vi "Front Panel Main Pange Horizontal Scroll Bar.vi"(8 "error in":errorcluster, 9 "Scrollbar Visibility":T1(ring)=enum."Off While Running", 11 "VI Ref In":refnum<vi>) -> (0 "error out":errorcluster, 3 "VI Ref Out":refnum<vi>)   [LabVIEW 2024]
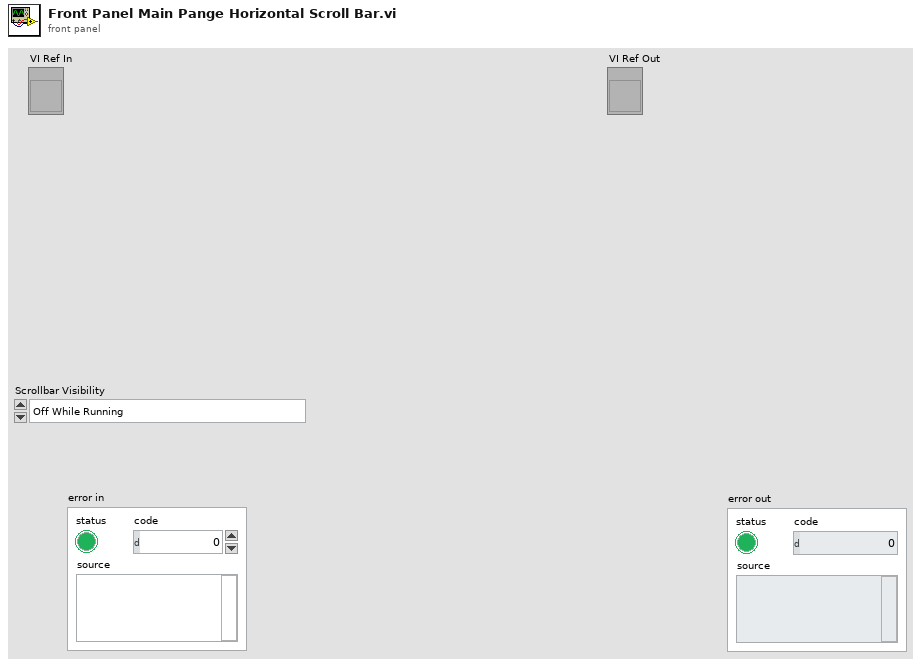
[diagram p1: front panel]
types:
  T1 = enum16{"Always On", "Always Off", "Off While Running"}
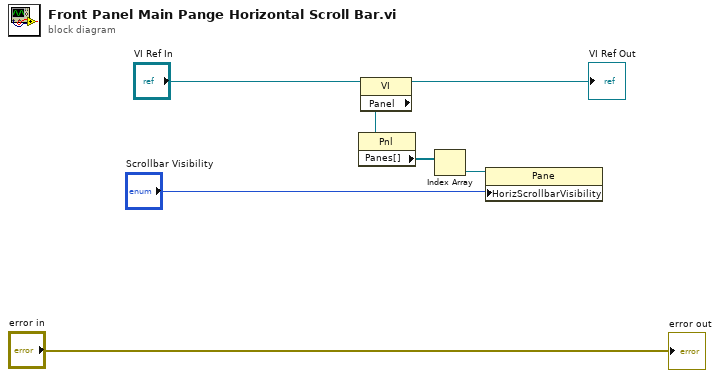
[diagram p0: block diagram]
diagram:
  n1 = property class="VI"(reference="VI Ref In") -> (reference out=→"VI Ref Out":refnum<vi>, "Panel"=w7:refnum<vi>)  [unwired: 1 in, 1 out]
  n2 = property class="Pnl"(reference=w7) -> ("Panes[]"=w6:refnum<vi>[])  [unwired: 1 in, 2 out]
  n3 = Index Array(array=w6) -> (element=w5:refnum<vi>)  [unwired: 1 in]
  n4 = property class="Pane"(reference=w5, "HorizScrollbarVisibility"="Scrollbar Visibility") -> ()  [unwired: 1 in, 2 out]
  "error out" <- "error in"
